vi "Close.vi"(6 "Timeout (180 s)":u32=180, 7 "Wait on reboot if needed (true)":bool=TRUE caption="Wait on restart if needed (T)", 8 "error in (no error)":errorcluster, 11 "RT Management in":refnum<class "RT Management.lvclass">) -> (0 "error out":errorcluster)   [LabVIEW 2015, in "RT Management.lvlib" / "RT Management.lvclass"]
doc: "Closes the File Transfer Session. Before doing so, the target is restarted if a restart has been deferred."
uses:
  RT Management.lvclass
  RT Management.lvclass/RT Management.ctl
  Get SysCfg Session.vi
  <vilib>/nisyscfg/Close (System).vi
  <vilib>/nisyscfg/nisyscfg.lvlib
panel:
  out "RT Management out":refnum<class "RT Management.lvclass">
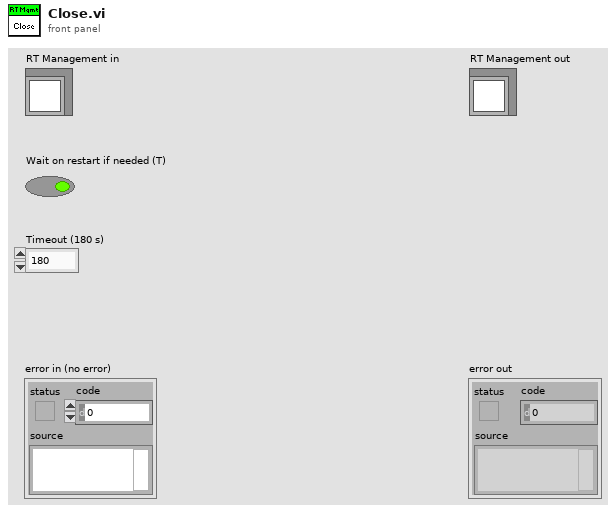
[diagram p1: front panel]
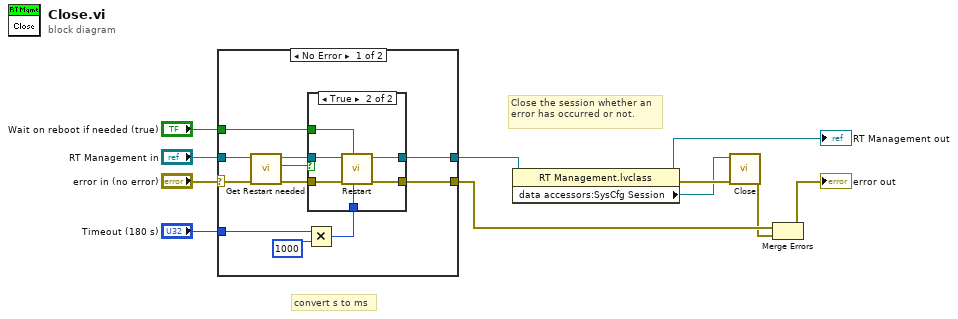
[diagram p0: block diagram]
diagram:
  # "convert s to ms"
  # "Close the session whether an error has occurred or not."
  n1 = case shown="No Error" "error in (no error)" {
    selector: "error in (no error)" -> [w22 w32]
    tunnel: [w15 w32] -> w4
    tunnel: [w16 w31] -> w7
    tunnel: "RT Management in" -> [w19 w31]
    tunnel: "Wait on reboot if needed (true)" -> [w17 _]
    tunnel: "Timeout (180 s)" -> [w14 _]
    frame No Error {
      n2 = call "Get Restart needed.vi"("error in (no error)"=w22, "RT Management Session in"=w19) -> ("error out"=w21:errorcluster, "Restart needed"=w18:bool, "RT Management Session out"=w20:refnum<class "RT Management.lvclass">)  [unwired: 7 in]
      n3 = Multiply(x=w14, y=u32 1000) -> (x*y=w12:u32)
      n4 = case shown="True" w18 {
        tunnel: [w23 w30] -> w15
        tunnel: w21 -> [w23 w29]
        tunnel: w20 -> [w24 w28]
        tunnel: [w24 w27] -> w16
        tunnel: w17 -> [_ w26]
        tunnel: w12 -> [_ w25]
        frame False {
        }
        frame True {
          n5 = call "Restart.vi"("Timeout msec (180000)"=w25, "Wait until complete (true)"=w26, "error in (no error)"=w29, "RT Management in"=w28) -> ("error out"=w30:errorcluster, "RT Management out"=w27:refnum<class "RT Management.lvclass">)  [unwired: 5 in]
        }
      }
    }
    frame Error {
    }
  }
  n6 = property class="RT Management.lvclass"(reference=w7) -> (reference out=→"RT Management out":refnum<class "RT Management.lvclass">, error out=w8:errorcluster, "data accessors:SysCfg Session"=w6:refnum<k21>)  [unwired: 1 in]
  n7 = call-poly <vilib>:"Close.vi"("error in (no error)"=w8, "Session in"=w6) -> ("error out"=w3:errorcluster)  [unwired: 9 in]
  n8 = Merge Errors(w4, w3) -> (→"error out":errorcluster)
